vi "VisualizeStatus.vi"() -> ()   [LabVIEW 2017, in "Visualization.lvlib" / "VisualizeStatus.lvclass"]
uses:
  VisualizeStatus.lvclass
  Framework/Bus_class/Bus.lvclass
  VisializeBase_class/Typedefs/VisualizeData.ctl
  VisializeBase_class/Typedefs/clVisualizeData.ctl
  Modules/EventPlugins/EventPluginBaseClass/TypeDefs/clEvtReportArray.ctl
  Modules/EventPlugins/EventPluginBaseClass/TypeDefs/clEvtReport.ctl
  Modules/EventPlugins/EventPluginBaseClass/TypeDefs/dblEvtSignalArray.ctl
  Modules/NetworkImpairmentModule/PublicAPI/Arguments/Broadcasts/dblNetworkTime.ctl
  Modules/NetworkImpairmentModule/PublicAPI/Arguments/Broadcasts/dblPktLoss.ctl
  Modules/FlagImpairModule/PublicAPI/Arguments/Broadcasts/ui32FlagImpairmentArray.ctl
  Framework/Bus_class/Broadcast/Typedefs/clDidInit.ctl
  Modules/EventModule/PublicAPI/Arguments/Broadcasts/clStatUpdate.ctl
  VisializeBase_class/Requests/clUserEventType.ctl
  <vilib>/event_ctls.llb/usereventprio.ctl
  <vilib>/Utility/miscctls.llb/LVStringsAndValuesArrayTypeDef_U8.ctl
  QMH/Typedefs/clEvtRptArray.ctl
  QMH/Typedefs/clPmuImpairRptArray.ctl
  QMH/Typedefs/clNetImpairmentTime.ctl
  QMH/Typedefs/clNetIPktLoss.ctl
  QMH/Typedefs/clFlagImpairArray.ctl
  QMH/Typedefs/clEvtRptSignal.ctl
  <vilib>/Utility/error.llb/Error Cluster From Error Code.vi
  <vilib>/ErrorRing/Error Ring.xnode
  VisializeBase_class/VisualizeBase_class.lvclass
  <userlib>/NIST/NISTErrorLib/NISTErrorLib.lvlib
  Framework/Bus_class/Bus_class.lvlib
  Modules/EventModule/EventModule.lvlib
  Modules/PmuImpairModule/PmuImpairModule.lvlib
  Modules/NetworkImpairmentModule/NetworkImpairmentModule.lvlib
  Modules/FlagImpairModule/FlagImpairModule.lvlib
  Modules/EventPlugins/EventPluginBaseClass/EventPluginBaseClass.lvclass
  VisualizeApp_class/VisualizeAppBase_class.lvclass
panel:
  in  "btnClear":bool
  out "Status Log":string
  in  "QueName":string="BaseVisQue"
  in  "Bus Number":u8(ring)
  out "ErrorArray":errorcluster[](array[cluster])
  in  "btnStop":bool
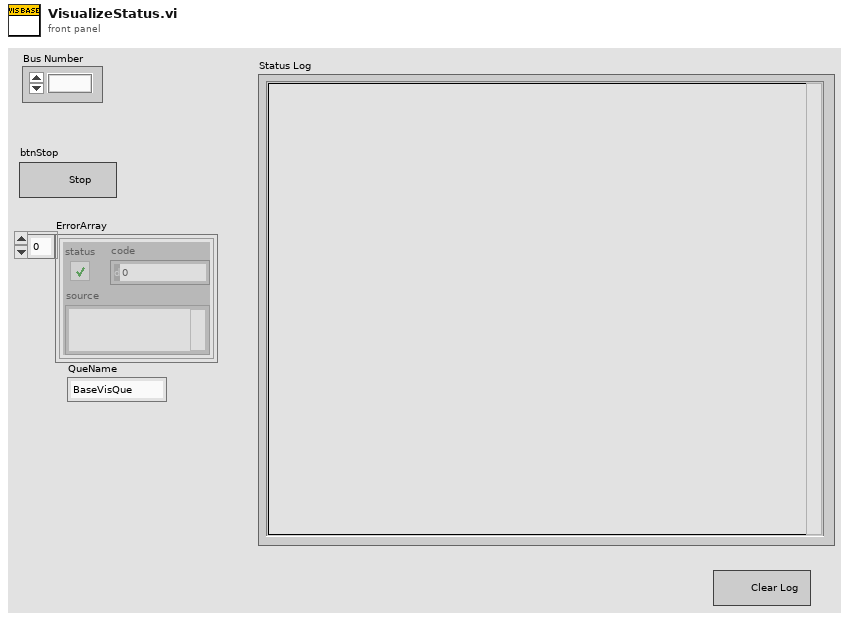
[diagram p1: front panel]
types:
  T1 = typedef "Visualization.lvlib/VisualizeBase_class.lvclass/VisualizeData.ctl" = T2[]
  T2 = typedef "Visualization.lvlib/VisualizeAppBase_class.lvclass/clVisualizeData.ctl" = cluster{"clEvtReportArray":T3, "dblEventSignalArray":T5, "clPmuImpairRptArray":T3, "dblNetworkTime":T6, "dblPktLoss":T7, "FlagImpairArray":T8, "TimeArray":dbl[]}
  T3 = typedef "EventPlugins.lvlib/EventPluginBaseClass.lvclass/clEvtReportArray.ctl" = T4[]
  T4 = typedef "EventPlugins.lvlib/EventPluginBaseClass.lvclass/clEvtReport.ctl" = cluster{"Timestamp":dbl, "Synx":cdb[], "Freq":dbl, "ROCOF":dbl, "ID":i16}
  T5 = typedef "EventPlugins.lvlib/EventPluginBaseClass.lvclass/dblEvtSignalArray.ctl" = dbl[][]
  T6 = typedef "NetworkImpairmentModule.lvlib/dblNetworkTime.ctl" = dbl[]
  T7 = typedef "NetworkImpairmentModule.lvlib/dblPktLoss.ctl" = dbl[]
  T8 = typedef "FlagImpairModule.lvlib/ui32FlagImpairmentArray.ctl" = u32[]
  T9 = typedef "Visualization.lvlib/VisualizeBase_class.lvclass/clRequestEvents.ctl" = cluster{"StopRequest":refnum<user-event>}
  T10 = typedef "Bus_class.lvlib/clBroadcastEvents.ctl" = cluster{"DidInit":refnum<user-event>, "DidStop":refnum<user-event>}
  T11 = typedef "EventModule.lvlib/clBroadcastEvents.ctl" = cluster{"DidInit":refnum<user-event>, "StatusUpdate":refnum<user-event>, "ErrorReport":refnum<user-event>, "DidStop":refnum<user-event>, "ReadEvtConfig":refnum<user-event>, "ReadTimeArray":refnum<user-event>, "ReadEvtParams":refnum<user-event>, "GetEvtReportArray":refnum<user-event>, "ReadPathToPlugin":refnum<user-event>, "GetEvtSignal":refnum<user-event>, "ReadBusNumber":refnum<user-event>}
  T12 = typedef "PmuImpairModule.lvlib/clBroadcastEvents.ctl" = cluster{"DidInit":refnum<user-event>, "StatusUpdate":refnum<user-event>, "ErrorReport":refnum<user-event>, "DidStop":refnum<user-event>, "ImpairConfig":refnum<user-event>, "ImpairParams":refnum<user-event>, "ImpairReports":refnum<user-event>, "PathToPlugin":refnum<user-event>, "BusNumber":refnum<user-event>}
  T13 = typedef "NetworkImpairmentModule.lvlib/clBroadcastEvents.ctl" = cluster{"DidInit":refnum<user-event>, "StatusUpdate":refnum<user-event>, "ErrorReport":refnum<user-event>, "DidStop":refnum<user-event>, "ReadNetImpParams":refnum<user-event>, "ReadLossThreshold":refnum<user-event>, "GetNetworkTime":refnum<user-event>, "GetPktLoss":refnum<user-event>, "ReadPathToPlugin":refnum<user-event>}
  T14 = typedef "FlagImpairModule.lvlib/clBroadcastEvents.ctl" = cluster{"DidInit":refnum<user-event>, "StatusUpdate":refnum<user-event>, "ErrorReport":refnum<user-event>, "DidStop":refnum<user-event>, "ReadFlagImpairConfig":refnum<user-event>, "ReadPluginINIFilePath":refnum<user-event>, "ReadFlagImpairParams":refnum<user-event>, "ReadTimeArray":refnum<user-event>, "GetFlagImpairment":refnum<user-event>}
  T15 = typedef "LVStringsAndValuesArrayTypeDef_U8.ctl" = cluster{"String":string, "Value":u8}[]
  T16 = typedef "Visualization.lvlib/VisualizeBase_class.lvclass/clEvtRptArray.ctl" = cluster{"BusIndex":i32, "clImpairReportArray":T3}
  T17 = typedef "EventModule.lvlib/clStatUpdate.ctl" = cluster{"Status":string}
  T18 = typedef "Visualization.lvlib/VisualizeBase_class.lvclass/clPmuImpairRptArray.ctl" = cluster{"BusIndex":i32, "clImpairReportArray":T3}
  T19 = typedef "Visualization.lvlib/VisualizeBase_class.lvclass/clNetImpairmentTime.ctl" = cluster{"BusIndex":i32, "clNetImpairTimeArray":T6}
  T20 = typedef "Visualization.lvlib/VisualizeBase_class.lvclass/clNetIPktLoss.ctl" = cluster{"BusIndex":i32, "clNetPktLoss":T7}
  T21 = typedef "Visualization.lvlib/VisualizeBase_class.lvclass/clFlagImpairArray.ctl" = cluster{"BusIndex":i32, "FlagImpairArray":T8}
  T22 = typedef "Visualization.lvlib/VisualizeBase_class.lvclass/clEvtRptSignal.ctl" = cluster{"BusIndex":i32, "dblEventSignalArray":T5}
  T23 = typedef "Visualization.lvlib/VisualizeBase_class.lvclass/clUserEventType.ctl" = cluster{"BusIndex":i8, "Data":variant}
  T24 = typedef "usereventprio.ctl" = enum32{"high priority", "normal priority"}
  T25 = typedef "Bus_class.lvlib/clDidInit.ctl" = cluster{"Bus":refnum<vi>, "Init?":bool}
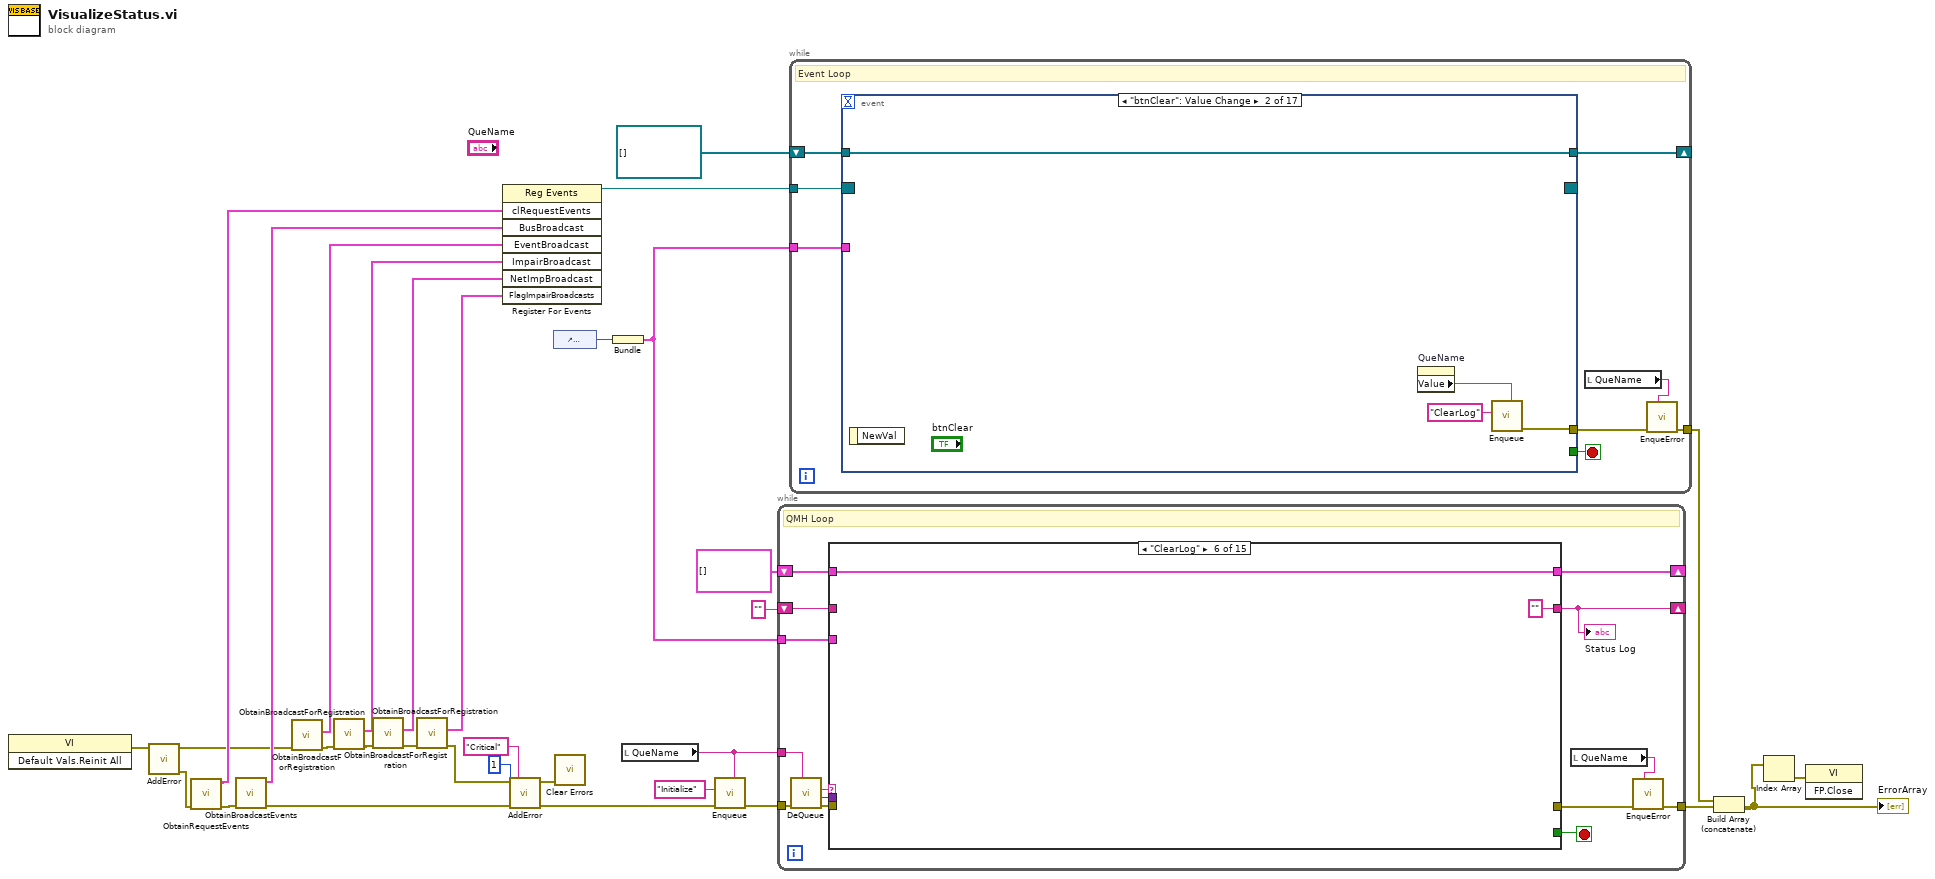
[diagram p0: block diagram]
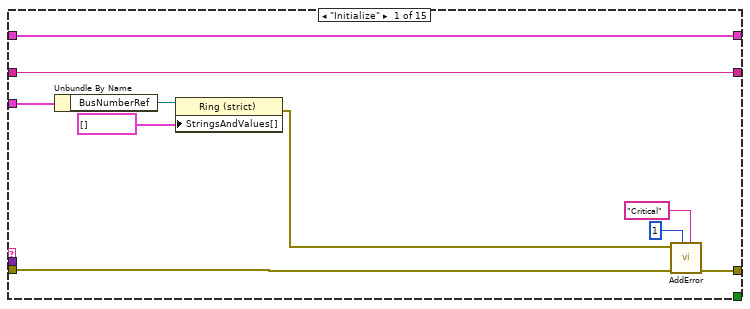
[diagram p2: hidden frame]
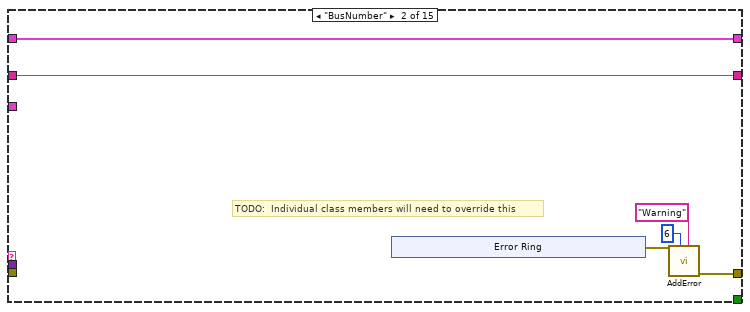
[diagram p3: hidden frame]
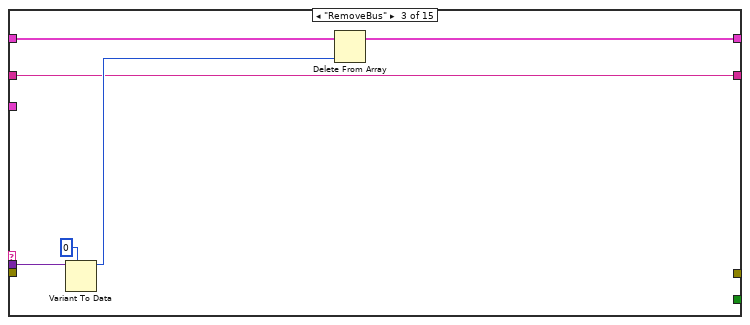
[diagram p4: hidden frame]
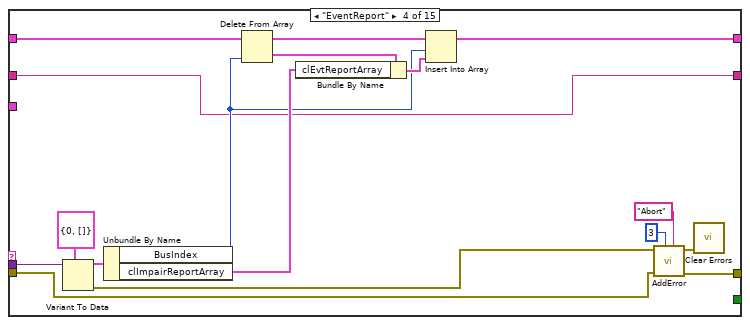
[diagram p5: hidden frame]
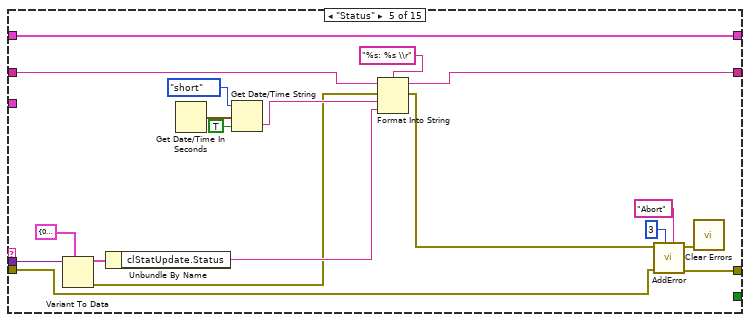
[diagram p6: hidden frame]
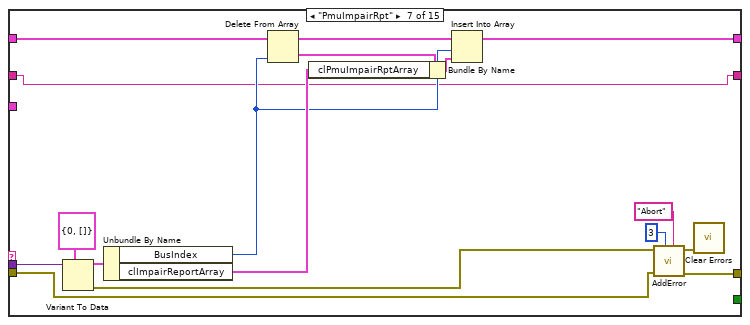
[diagram p7: hidden frame]
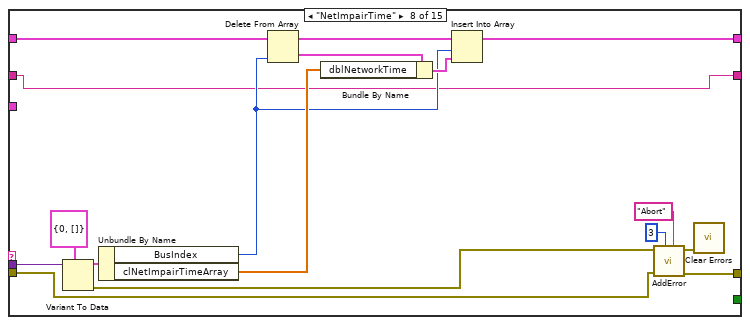
[diagram p8: hidden frame]
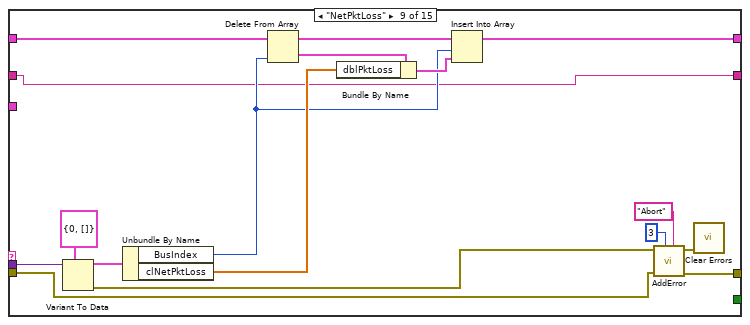
[diagram p9: hidden frame]
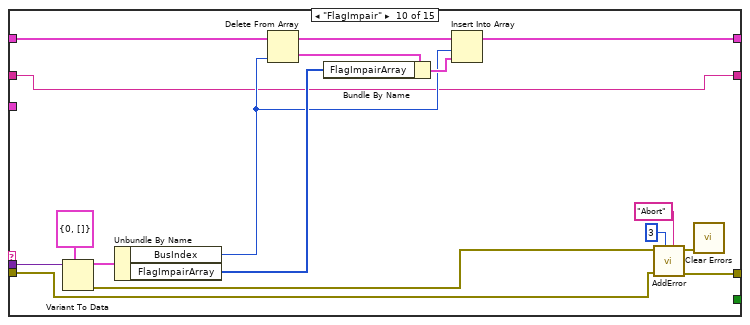
[diagram p10: hidden frame]
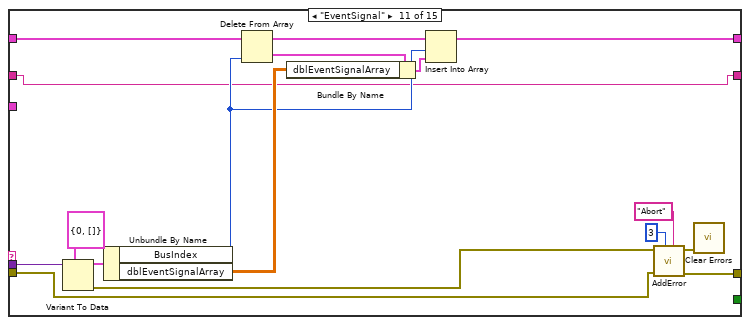
[diagram p11: hidden frame]
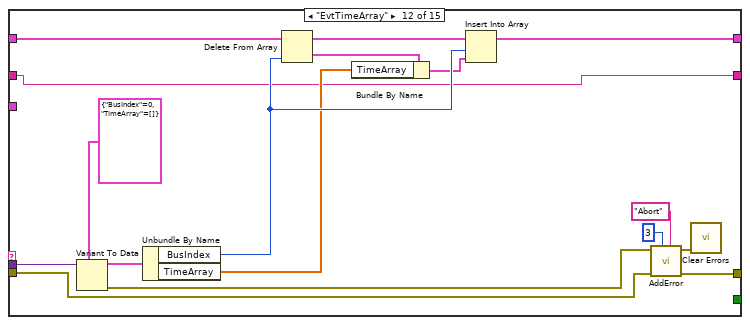
[diagram p12: hidden frame]
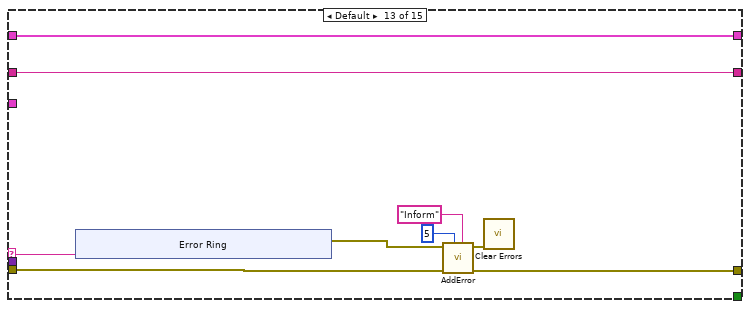
[diagram p13: hidden frame]
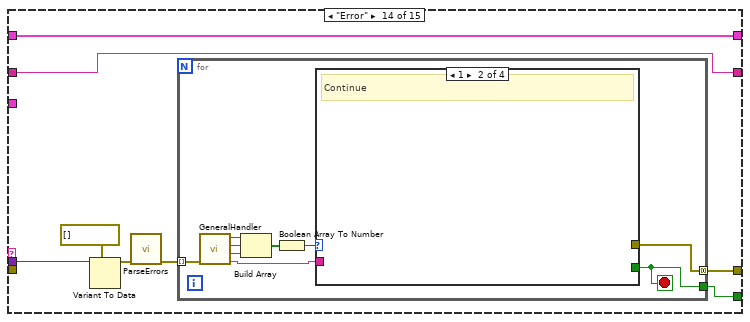
[diagram p14: hidden frame]
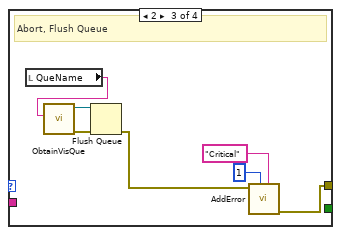
[diagram p16: hidden frame]
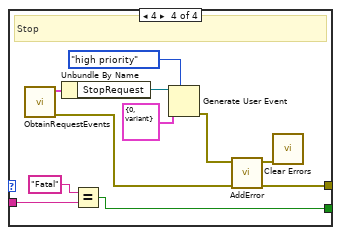
[diagram p17: hidden frame]
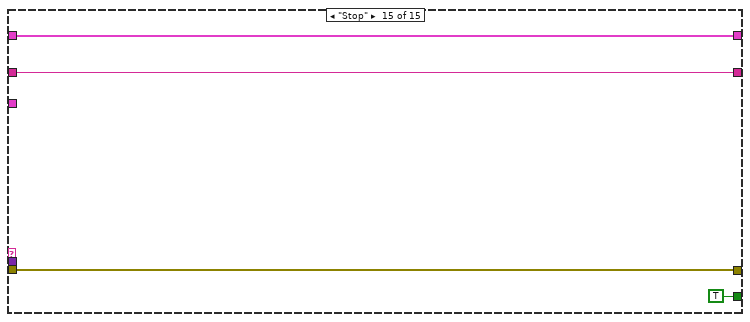
[diagram p18: hidden frame]
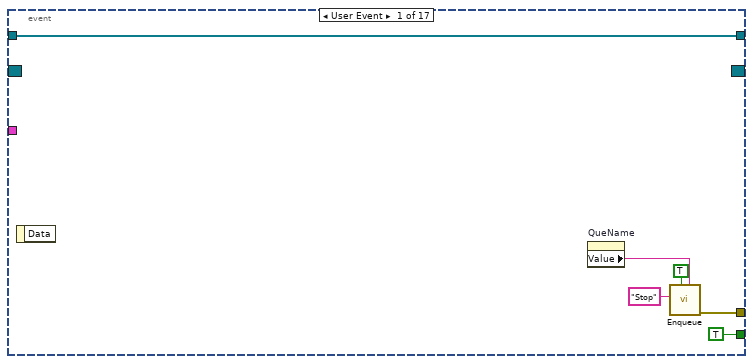
[diagram p19: hidden frame]
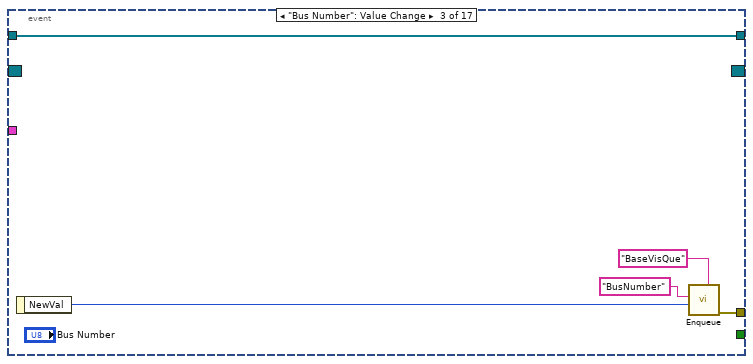
[diagram p20: hidden frame]
diagram:
  n1 = invoke class="VI" method="Default Vals.Reinit All"() -> (error out=w22:errorcluster)  [unwired: 3 in, 2 out]
  n2 = call <userlib>:"AddError.vi"("error in (no error)"=w22) -> ("ErrorArray"=w21:errorcluster[], "error out"=w13:errorcluster)  [unwired: 9 in]
  n3 = call "ObtainRequestEvents.vi"("Error"=w21) -> ("Error"=w26:errorcluster[], "clRequestEvents"=w30:T9)  [unwired: 9 in]
  n4 = call "ObtainBroadcastEvents.vi"("ErrorArray"=w26) -> ("ErrorArray"=w12:errorcluster[], "BusBroadcast"=w25:T10)  [unwired: 9 in]
  n5 = call "ObtainBroadcastForRegistration.vi"("error in (no error)"=w13) -> ("error out"=w16:errorcluster, "EventBroadcast"=w20:T11)  [unwired: 9 in]
  n6 = call "ObtainBroadcastForRegistration.vi"("error in (no error)"=w16) -> ("error out"=w15:errorcluster, "ImpairBroadcast"=w19:T12)  [unwired: 9 in]
  n7 = call "ObtainBroadcastForRegistration.vi"("error in (no error)"=w15) -> ("error out"=w14:errorcluster, "NetImpBroadcast"=w18:T13)  [unwired: 9 in]
  n8 = call "ObtainBroadcastForRegistration.vi"("error in (no error)"=w14) -> ("error out"=w11:errorcluster, "FlagImpairBroadcasts"=w17:T14)  [unwired: 9 in]
  n9 = register-events(w30, w25, w20, w19, w18, w17) -> (reference out=w29:refnum<event-registration>)  [unwired: 2 in, 1 out]
  n10 = call <userlib>:"AddError.vi"("Severity"="Critical" ("String"), "Priority"=u8 1, "ErrorArray"=w12, "error in (no error)"=w11) -> ("ErrorArray"=w8:errorcluster[], "error out"=w5:errorcluster)  [unwired: 6 in]
  n11 = control-ref of="BusNumberRef"() -> (w24:refnum<vi>)
  n12 = call <vilib>:"Clear Errors.vi"("error in (no error)"=w5) -> ()  [unwired: 5 in, 2 out]
  n13 = Bundle("BusNumberRef"=w24) -> (w6:cluster{"BusNumberRef":refnum<vi>})  [unwired: 1 in]
  n14 = local read "QueName"() -> (w4:string)
  n15 = call "Enqueue.vi"("QueName"=w4, "Error"=w8, "Message"="Initialize") -> ("Error"=w31:errorcluster[])  [unwired: 8 in]
  n16 = while {
    tunnel: w31 -> [w46]
    tunnel: [w40] -> w28
    tunnel: w6 -> [w39]
    shift-right: [w37] -> _
    shift-left: T1 [] ("VisualizeData") -> [w38]
    tunnel: w4 -> [w35]
    shift-right: [w33] -> _
    shift-left: "" -> [w34]
    stop <- w41 stop-if-true
    # "QMH Loop"
    n17 = call "DeQueue.vi"("QueName"=w35, "Error"=w46) -> ("Error"=w43:errorcluster[], "Data"=w44:variant, "Message"=w45:string)  [unwired: 7 in]
    n18 = case shown="\"ClearLog\"" w45 {
      selector: w45 -> [_ _ _ _ _ _ _ _ _ _ _ _ w222 _ _]
      tunnel: w44 -> [_ _ w73 w90 w109 _ w128 w145 w162 w179 w196 w204 _ w237 _]
      tunnel: w43 -> [w53 _ _ w75 w103 _ w113 w130 w147 w164 w181 w198 w220 _ w267]
      tunnel: [w52 w62 _ w80 w107 _ w118 w135 w152 w169 w186 w200 w219 w233 w267] -> w42
      tunnel: [_ _ _ _ _ _ _ _ _ _ _ _ _ w232 TRUE] -> w41
      tunnel: w39 -> [w56 _ _ _ _ _ _ _ _ _ _ _ _ _ _]
      tunnel: w38 -> [w48 w58 w71 w86 w102 w110 w124 w141 w158 w175 w192 w206 w215 w231 w266]
      tunnel: [w48 w58 w70 w87 w102 w110 w125 w142 w159 w176 w193 w205 w215 w231 w266] -> w37
      tunnel: w34 -> [w47 w57 w68 w74 w96 _ w112 w129 w146 w163 w180 w197 w214 w230 w265]
      tunnel: [w47 w57 w68 w74 w95 "" w112 w129 w146 w163 w180 w197 w214 w230 w265] -> w33
      frame "Initialize" {
        n19 = Unbundle By Name(w56) -> ("BusNumberRef"=w55:refnum<vi>)
        n20 = property class="Ring (strict)"(reference=w55, "StringsAndValues[]"=T15 [] ("Strings And Values []")) -> (error out=w51:errorcluster)  [unwired: 1 in, 1 out]
        n21 = call <userlib>:"AddError.vi"("Severity"="Critical" ("String"), "Priority"=u8 1, "ErrorArray"=w53, "error in (no error)"=w51) -> ("ErrorArray"=w52:errorcluster[])  [unwired: 6 in, 1 out]
      }
      frame "BusNumber" {
        # "TODO:  Individual class members will need to override this"
        n22 = xnode "Error Ring"() -> ("error out"=w61:errorcluster)
        n23 = call <userlib>:"AddError.vi"("Severity"="Warning" ("String"), "Priority"=u8 6, "error in (no error)"=w61) -> ("ErrorArray"=w62:errorcluster[])  [unwired: 7 in, 1 out]
      }
      frame "RemoveBus" {
        n24 = Variant To Data(type=0, Variant=w73) -> (data=w69:i32)  [unwired: 1 in, 1 out]
        n25 = Delete From Array(array=w71, index=w69) -> (array with subset deleted=w70:T1)  [unwired: 1 in, 1 out]
      }
      frame "EventReport" {
        n26 = Variant To Data(type=T16 {"BusIndex"=0, "clImpairReportArray"=[]} ("clEvtReportArray"), Variant=w90) -> (data=w88:T16, error out=w79:errorcluster)  [unwired: 1 in]
        n27 = Unbundle By Name(w88) -> ("BusIndex"=w81:i32, "clImpairReportArray"=w83:T3)
        n28 = Delete From Array(array=w86, index=w81) -> (deleted portion=w84:T2, array with subset deleted=w85:T1)  [unwired: 1 in]
        n29 = Bundle By Name(cluster=w84, "clEvtReportArray"=w83) -> (w82:T2)
        n30 = Insert Into Array(array=w85, index=w81, new element=w82) -> (w87:T1)
        n31 = call <userlib>:"AddError.vi"("Severity"="Abort" ("String"), "Priority"=u8 3, "ErrorArray"=w75, "error in (no error)"=w79) -> ("ErrorArray"=w80:errorcluster[], "error out"=w78:errorcluster)  [unwired: 6 in]
        n32 = call <vilib>:"Clear Errors.vi"("error in (no error)"=w78) -> ()  [unwired: 5 in, 2 out]
      }
      frame "Status" {
        n33 = Variant To Data(type=cluster{i32, "clStatUpdate":T17} {0, "clStatUpdate"={"Status"=""}} ("output cluster"), Variant=w109) -> (data=w108:cluster{i32, "clStatUpdate":T17}, error out=w93:errorcluster)  [unwired: 1 in]
        n34 = Unbundle By Name(w108) -> ("clStatUpdate.Status"=w94:string)
        n35 = Get Date/Time In Seconds() -> (seconds since 1Jan1904=w98:timestamp)
        n36 = Get Date/Time String(date format (0)=enum16{"short", "long", "abbreviated"}."short", seconds (now)=w98, want seconds? (F)=TRUE) -> (time string=w101:string)  [unwired: 1 out]
        n37 = Format Into String(format string="%s: %s \\r", initial string=w96, error in=w93, w101, w94) -> (resulting string=w95:string, error out=w92:errorcluster)
        n38 = call <userlib>:"AddError.vi"("Severity"="Abort" ("String"), "Priority"=u8 3, "ErrorArray"=w103, "error in (no error)"=w92) -> ("ErrorArray"=w107:errorcluster[], "error out"=w106:errorcluster)  [unwired: 6 in]
        n39 = call <vilib>:"Clear Errors.vi"("error in (no error)"=w106) -> ()  [unwired: 5 in, 2 out]
      }
      frame "ClearLog" {
      }
      frame "PmuImpairRpt" {
        n40 = Variant To Data(type=T18 {"BusIndex"=0, "clImpairReportArray"=[]} ("clImpairReportArray"), Variant=w128) -> (data=w126:T18, error out=w117:errorcluster)  [unwired: 1 in]
        n41 = Unbundle By Name(w126) -> ("BusIndex"=w119:i32, "clImpairReportArray"=w121:T3)
        n42 = Delete From Array(array=w124, index=w119) -> (deleted portion=w122:T2, array with subset deleted=w123:T1)  [unwired: 1 in]
        n43 = Bundle By Name(cluster=w122, "clPmuImpairRptArray"=w121) -> (w120:T2)
        n44 = Insert Into Array(array=w123, index=w119, new element=w120) -> (w125:T1)
        n45 = call <userlib>:"AddError.vi"("Severity"="Abort" ("String"), "Priority"=u8 3, "ErrorArray"=w113, "error in (no error)"=w117) -> ("ErrorArray"=w118:errorcluster[], "error out"=w116:errorcluster)  [unwired: 6 in]
        n46 = call <vilib>:"Clear Errors.vi"("error in (no error)"=w116) -> ()  [unwired: 5 in, 2 out]
      }
      frame "NetImpairTime" {
        n47 = Variant To Data(type=T19 {"BusIndex"=0, "clNetImpairTimeArray"=[]} ("clImpairReportArray"), Variant=w145) -> (data=w143:T19, error out=w134:errorcluster)  [unwired: 1 in]
        n48 = Unbundle By Name(w143) -> ("BusIndex"=w136:i32, "clNetImpairTimeArray"=w138:T6)
        n49 = Delete From Array(array=w141, index=w136) -> (deleted portion=w139:T2, array with subset deleted=w140:T1)  [unwired: 1 in]
        n50 = Bundle By Name(cluster=w139, "dblNetworkTime"=w138) -> (w137:T2)
        n51 = Insert Into Array(array=w140, index=w136, new element=w137) -> (w142:T1)
        n52 = call <userlib>:"AddError.vi"("Severity"="Abort" ("String"), "Priority"=u8 3, "ErrorArray"=w130, "error in (no error)"=w134) -> ("ErrorArray"=w135:errorcluster[], "error out"=w133:errorcluster)  [unwired: 6 in]
        n53 = call <vilib>:"Clear Errors.vi"("error in (no error)"=w133) -> ()  [unwired: 5 in, 2 out]
      }
      frame "NetPktLoss" {
        n54 = Variant To Data(type=T20 {"BusIndex"=0, "clNetPktLoss"=[]} ("clNetPktLoss"), Variant=w162) -> (data=w160:T20, error out=w151:errorcluster)  [unwired: 1 in]
        n55 = Unbundle By Name(w160) -> ("BusIndex"=w153:i32, "clNetPktLoss"=w155:T7)
        n56 = Delete From Array(array=w158, index=w153) -> (deleted portion=w156:T2, array with subset deleted=w157:T1)  [unwired: 1 in]
        n57 = Bundle By Name(cluster=w156, "dblPktLoss"=w155) -> (w154:T2)
        n58 = Insert Into Array(array=w157, index=w153, new element=w154) -> (w159:T1)
        n59 = call <userlib>:"AddError.vi"("Severity"="Abort" ("String"), "Priority"=u8 3, "ErrorArray"=w147, "error in (no error)"=w151) -> ("ErrorArray"=w152:errorcluster[], "error out"=w150:errorcluster)  [unwired: 6 in]
        n60 = call <vilib>:"Clear Errors.vi"("error in (no error)"=w150) -> ()  [unwired: 5 in, 2 out]
      }
      frame "FlagImpair" {
        n61 = Variant To Data(type=T21 {"BusIndex"=0, "FlagImpairArray"=[]} ("clFlagImpairArray"), Variant=w179) -> (data=w177:T21, error out=w168:errorcluster)  [unwired: 1 in]
        n62 = Unbundle By Name(w177) -> ("BusIndex"=w170:i32, "FlagImpairArray"=w172:T8)
        n63 = Delete From Array(array=w175, index=w170) -> (deleted portion=w173:T2, array with subset deleted=w174:T1)  [unwired: 1 in]
        n64 = Bundle By Name(cluster=w173, "FlagImpairArray"=w172) -> (w171:T2)
        n65 = Insert Into Array(array=w174, index=w170, new element=w171) -> (w176:T1)
        n66 = call <userlib>:"AddError.vi"("Severity"="Abort" ("String"), "Priority"=u8 3, "ErrorArray"=w164, "error in (no error)"=w168) -> ("ErrorArray"=w169:errorcluster[], "error out"=w167:errorcluster)  [unwired: 6 in]
        n67 = call <vilib>:"Clear Errors.vi"("error in (no error)"=w167) -> ()  [unwired: 5 in, 2 out]
      }
      frame "EventSignal" {
        n68 = Variant To Data(type=T22 {"BusIndex"=0, "dblEventSignalArray"=[]} ("clEvtReportArray"), Variant=w196) -> (data=w194:T22, error out=w185:errorcluster)  [unwired: 1 in]
        n69 = Unbundle By Name(w194) -> ("BusIndex"=w187:i32, "dblEventSignalArray"=w189:T5)
        n70 = Delete From Array(array=w192, index=w187) -> (deleted portion=w190:T2, array with subset deleted=w191:T1)  [unwired: 1 in]
        n71 = Bundle By Name(cluster=w190, "dblEventSignalArray"=w189) -> (w188:T2)
        n72 = Insert Into Array(array=w191, index=w187, new element=w188) -> (w193:T1)
        n73 = call <userlib>:"AddError.vi"("Severity"="Abort" ("String"), "Priority"=u8 3, "ErrorArray"=w181, "error in (no error)"=w185) -> ("ErrorArray"=w186:errorcluster[], "error out"=w184:errorcluster)  [unwired: 6 in]
        n74 = call <vilib>:"Clear Errors.vi"("error in (no error)"=w184) -> ()  [unwired: 5 in, 2 out]
      }
      frame "EvtTimeArray" {
        n75 = Variant To Data(type=cluster{"BusIndex":i32, "TimeArray":dbl[]} {"BusIndex"=0, "TimeArray"=[]} ("cluster"), Variant=w204) -> (data=w207:cluster{"BusIndex":i32, "TimeArray":dbl[]}, error out=w199:errorcluster)  [unwired: 1 in]
        n76 = Unbundle By Name(w207) -> ("BusIndex"=w212:i32, "TimeArray"=w210:dbl[])
        n77 = Delete From Array(array=w206, index=w212) -> (deleted portion=w209:T2, array with subset deleted=w208:T1)  [unwired: 1 in]
        n78 = Bundle By Name(cluster=w209, "TimeArray"=w210) -> (w211:T2)
        n79 = Insert Into Array(array=w208, index=w212, new element=w211) -> (w205:T1)
        n80 = call <userlib>:"AddError.vi"("Severity"="Abort" ("String"), "Priority"=u8 3, "ErrorArray"=w198, "error in (no error)"=w199) -> ("ErrorArray"=w200:errorcluster[], "error out"=w201:errorcluster)  [unwired: 6 in]
        n81 = call <vilib>:"Clear Errors.vi"("error in (no error)"=w201) -> ()  [unwired: 5 in, 2 out]
      }
      frame Default {
        n82 = xnode "Error Ring"("parameter 0"=w222) -> ("error out"=w221:errorcluster)
        n83 = call <userlib>:"AddError.vi"("Severity"="Inform" ("String"), "Priority"=u8 5, "ErrorArray"=w220, "error in (no error)"=w221) -> ("ErrorArray"=w219:errorcluster[], "error out"=w218:errorcluster)  [unwired: 6 in]
        n84 = call <vilib>:"Clear Errors.vi"("error in (no error)"=w218) -> ()  [unwired: 5 in, 2 out]
      }
      frame "Error" {
        n85 = Variant To Data(type=errorcluster[] [], Variant=w237) -> (data=w235:errorcluster[])  [unwired: 1 in, 1 out]
        n86 = call <userlib>:"ParseErrors.vi"("ErrorArray"=w235) -> ("ErrorArray"=w234:errorcluster[])  [unwired: 8 in, 2 out]
        n87 = for {
          tunnel: w234 -> [w246] mode=indexing
          tunnel: [w240] -> w233 mode=concatenating
          tunnel: [w238] -> w232
          stop <- w238 stop-if-true
          n88 = call <userlib>:"GeneralHandler.vi"("error in (no error)"=w246) -> ("Severity"=w239:string, "Stop"=w243:bool, "Abort"=w244:bool, "Continue"=w245:bool)  [unwired: 7 in]
          n89 = Build Array(w245, w244, w243) -> (w242:bool[])
          n90 = Boolean Array To Number(Boolean array=w242) -> (number=w241:u32)
          n91 = case shown="1" w241 {
            tunnel: [_ _ w251 w262] -> w240
            tunnel: w239 -> [_ _ _ w256]
            tunnel: [_ _ _ w254] -> w238
            frame 0, Default {
              # "No Dialog"
            }
            frame 1 {
              # "Continue"
            }
            frame 2 {
              # "Abort, Flush Queue"
              n92 = local read "QueName"() -> (w247:string)
              n93 = call "ObtainVisQue.vi"("QueName"=w247) -> ("error out"=w253:errorcluster, "queue out"=w252:refnum<queue>)  [unwired: 9 in]
              n94 = Flush Queue(queue=w252, error in (no error)=w253) -> (error out=w250:errorcluster)  [unwired: 2 out]
              n95 = call <userlib>:"AddError.vi"("Severity"="Critical" ("String"), "Priority"=u8 1, "error in (no error)"=w250) -> ("ErrorArray"=w251:errorcluster[])  [unwired: 7 in, 1 out]
            }
            frame 4 {
              # "Stop"
              n96 = call "ObtainRequestEvents.vi"() -> ("Error"=w260:errorcluster[], "clRequestEvents"=w264:T9)  [unwired: 10 in]
              n97 = Unbundle By Name(w264) -> ("StopRequest"=w263:refnum<user-event>)
              n98 = Equal?(x="Fatal", y=w256) -> (x = y?=w254:bool)
              n99 = Generate User Event(priority (normal)=usereventprio."high priority", user event=w263, event data cluster=T23 {"BusIndex"=0, "Data"=variant} ("event data")) -> (error out=w261:errorcluster)  [unwired: 1 in, 1 out]
              n100 = call <userlib>:"AddError.vi"("ErrorArray"=w260, "error in (no error)"=w261) -> ("ErrorArray"=w262:errorcluster[], "error out"=w257:errorcluster)  [unwired: 8 in]
              n101 = call <vilib>:"Clear Errors.vi"("error in (no error)"=w257) -> ()  [unwired: 5 in, 2 out]
            }
          }
        }
      }
      frame "Stop" {
      }
    }
    "Status Log" <- w33
    n102 = local read "QueName"() -> (w36:string)
    n103 = call "EnqueError.vi"("QueName"=w36, "Error"=w42) -> ("Error"=w40:errorcluster[])  [unwired: 9 in]
  }
  n104 = while {
    tunnel: w29 -> [w276]
    tunnel: [w273] -> w27
    tunnel: w6 -> [w272]
    shift-right: [w270] -> _
    shift-left: refnum<class "Bus.lvclass">[] [] -> [w271]
    stop <- w275 stop-if-true
    # "Event Loop"
    n105 = event shown="[1] \"btnClear\": Value Change" {
      selector: w276 -> [_ _ _ _ _ _ _ _ _ _ _ _ _ _ _ _ _]
      dyn-events: [_ _ _ w300 _ _ _ _ _ _ _ _ _ _ _ _ _] -> _
      timeout: _ -> [_ _ _ _ _ _ _ _ _ _ _ _ _ _ _ _ _]
      tunnel: [TRUE _ _ _ _ _ _ _ _ _ _ _ _ _ _ _ _] -> w275
      tunnel: [w281 w285 w291 w303 w321 w327 w355 w383 w411 w439 w468 w491 w514 w537 w560 w583 w610] -> w274
      tunnel: w272 -> [_ _ _ w313 w325 _ _ _ _ _ _ _ _ _ _ _ _]
      tunnel: w271 -> [w278 w286 w288 w312 w324 w328 w356 w384 w412 w440 w471 w494 w517 w540 w563 w586 w604]
      tunnel: [w278 w286 w288 w309 w323 w326 w354 w382 w410 w438 w466 w489 w512 w535 w558 w581 w604] -> w270
      event User Event {
        n106 = event-data() -> ()  [unwired: 1 in, 1 out]
        n107 = property on="QueName" class="Str"() -> ("Value"=w277:string)  [unwired: 2 in, 2 out]
        n108 = call "Enqueue.vi"("QueName"=w277, "Priority? (F)"=TRUE, "Message"="Stop") -> ("Error"=w281:errorcluster[])  [unwired: 8 in]
      }
      event "btnClear": Value Change {
        n109 = event-data() -> ()  [unwired: 1 in, 1 out]
        n110 = property on="QueName" class="Str"() -> ("Value"=w284:string)  [unwired: 2 in, 2 out]
        n111 = call "Enqueue.vi"("QueName"=w284, "Message"="ClearLog") -> ("Error"=w285:errorcluster[])  [unwired: 9 in]
      }
      event "Bus Number": Value Change {
        n112 = event-data() -> ("NewVal"=w290:u8)  [unwired: 1 in]
        n113 = call "Enqueue.vi"("QueName"="BaseVisQue", "Data"=w290, "Message"="BusNumber") -> ("Error"=w291:errorcluster[])  [unwired: 8 in]
      }
      event User Event {
        n114 = event-data() -> ("Data"=w316:variant)  [unwired: 1 in]
        n115 = Unbundle By Name(w313) -> ("BusNumberRef"=w311:refnum<vi>)
        n116 = Variant To Data(type=T25 {"Bus"=refnum, "Init?"=FALSE} ("clBusDidInit"), Variant=w316) -> (data=w314:T25)  [unwired: 1 in, 1 out]
        n117 = Unbundle By Name(w314) -> ("Bus"=w310:refnum<vi>)
        n118 = call "AddBus.vi"("BusRef"=w310, "BusNumberRef"=w311, "BusArray"=w312) -> ("BusArray"=w309:refnum<class "Bus.lvclass">[])  [unwired: 8 in]
        n119 = call "ObtainRequestEvents.vi"() -> ("Error"=w295:errorcluster[], "clRequestEvents"=w293:T9)  [unwired: 10 in]
        n120 = call "ObtainBroadcastEvents.vi"("ErrorArray"=w295) -> ("ErrorArray"=w294:errorcluster[], "BusBroadcast"=w292:T10)  [unwired: 9 in]
        n121 = call "ObtainBroadcastForRegistration.vi"() -> ("error out"=w308:errorcluster, "EventBroadcast"=w299:T11)  [unwired: 10 in]
        n122 = call "ObtainBroadcastForRegistration.vi"("error in (no error)"=w308) -> ("error out"=w307:errorcluster, "ImpairBroadcast"=w298:T12)  [unwired: 9 in]
        n123 = call "ObtainBroadcastForRegistration.vi"("error in (no error)"=w307) -> ("error out"=w306:errorcluster, "NetImpBroadcast"=w297:T13)  [unwired: 9 in]
        n124 = call "ObtainBroadcastForRegistration.vi"("error in (no error)"=w306) -> ("error out"=w301:errorcluster, "FlagImpairBroadcasts"=w296:T14)  [unwired: 9 in]
        n125 = register-events(w293, w292, w299, w298, w297, w296) -> (reference out=w300:refnum<event-registration>)  [unwired: 2 in, 1 out]
        n126 = call <userlib>:"AddError.vi"("Severity"="Critical" ("String"), "Priority"=u8 1, "ErrorArray"=w294, "error in (no error)"=w301) -> ("ErrorArray"=w303:errorcluster[], "error out"=w302:errorcluster)  [unwired: 6 in]
        n127 = call <vilib>:"Clear Errors.vi"("error in (no error)"=w302) -> ()  [unwired: 5 in, 2 out]
      }
      event User Event {
        n128 = event-data() -> ("BusNumber"=w318:i8)  [unwired: 1 in]
        n129 = Unbundle By Name(w325) -> ("BusNumberRef"=w322:refnum<vi>)
        n130 = call "RemoveBus.vi"("BusArray"=w324, "BusNumberRef"=w322, "BusNumber"=w318) -> ("BusArray"=w323:refnum<class "Bus.lvclass">[], "BusIndex"=w320:i32)  [unwired: 6 in]
        n131 = call "Enqueue.vi"("QueName"="BaseVisQue", "Data"=w320, "Message"="RemoveBus") -> ("Error"=w321:errorcluster[])  [unwired: 8 in]
      }
      event User Event {
        w329 = FALSE  # Enabled?
        n132 = event-data() -> ("ModuleID"=w331:i32, "Data"=w330:variant)  [unwired: 1 in]
        n133 = case shown="True" w329 {
          tunnel: [w332 w348] -> w326
          tunnel: w328 -> [w332 w348]
          tunnel: w331 -> [_ w345]
          tunnel: w330 -> [_ w347]
          tunnel: [_ w335] -> w327
          frame False {
          }
          frame True {
            n134 = Variant To Data(type=dbl[] [], Variant=w347) -> (data=w344:dbl[], error out=w340:errorcluster)  [unwired: 1 in]
            n135 = for {
              tunnel: w348 -> [w353] mode=indexing
              tunnel: w345 -> [w351]
              tunnel: [w349] -> w334
              i -> [w349]
              stop <- w350 stop-if-true
              # "Find Bus Index"
              n136 = property class="Bus.lvclass"(reference=w353) -> ("Accessors:EventModuleID"=w352:i32)  [unwired: 1 in, 2 out]
              n137 = Equal?(x=w352, y=w351) -> (x = y?=w350:bool)
            }
            n138 = call <userlib>:"AddError.vi"("Severity"="Critical" ("String"), "Priority"=u8 1, "error in (no error)"=w340) -> ("ErrorArray"=w336:errorcluster[], "error out"=w339:errorcluster)  [unwired: 7 in]
            n139 = call <vilib>:"Clear Errors.vi"("error in (no error)"=w339) -> ()  [unwired: 5 in, 2 out]
            n140 = Bundle(w334, w344) -> (w343:cluster{i32, dbl[]})  [unwired: 1 in]
            n141 = To Variant(anything=w343) -> (Variant=w342:variant)
            n142 = call "Enqueue.vi"("QueName"="BaseVisQue", "Error"=w336, "Data"=w342, "Message"="EvtTimeArray") -> ("Error"=w335:errorcluster[])  [unwired: 7 in]
          }
        }
      }
      event User Event {
        w357 = TRUE  # Enabled?
        n143 = event-data() -> ("ModuleID"=w359:i32, "Data"=w358:variant)  [unwired: 1 in]
        n144 = case shown="True" w357 {
          tunnel: [w360 w376] -> w354
          tunnel: w356 -> [w360 w376]
          tunnel: w359 -> [_ w374]
          tunnel: w358 -> [_ w375]
          tunnel: [_ w364] -> w355
          frame False {
          }
          frame True {
            n145 = Variant To Data(type=T17 {"Status"=""} ("clStatUpdate"), Variant=w375) -> (data=w373:T17, error out=w369:errorcluster)  [unwired: 1 in]
            n146 = for {
              tunnel: w376 -> [w381] mode=indexing
              tunnel: w374 -> [w379]
              tunnel: [w377] -> w363
              i -> [w377]
              stop <- w378 stop-if-true
              # "Find Bus Index"
              n147 = property class="Bus.lvclass"(reference=w381) -> ("Accessors:EventModuleID"=w380:i32)  [unwired: 1 in, 2 out]
              n148 = Equal?(x=w380, y=w379) -> (x = y?=w378:bool)
            }
            n149 = call <userlib>:"AddError.vi"("Severity"="Critical" ("String"), "Priority"=u8 1, "error in (no error)"=w369) -> ("ErrorArray"=w365:errorcluster[], "error out"=w368:errorcluster)  [unwired: 7 in]
            n150 = call <vilib>:"Clear Errors.vi"("error in (no error)"=w368) -> ()  [unwired: 5 in, 2 out]
            n151 = Bundle(w363, "clStatUpdate"=w373) -> (w372:cluster{i32, "clStatUpdate":T17})  [unwired: 1 in]
            n152 = To Variant(anything=w372) -> (Variant=w371:variant)
            n153 = call "Enqueue.vi"("QueName"="BaseVisQue", "Error"=w365, "Data"=w371, "Message"="Status") -> ("Error"=w364:errorcluster[])  [unwired: 7 in]
          }
        }
      }
      event User Event {
        w385 = TRUE  # Enabled?
        n154 = event-data() -> ("ModuleID"=w387:i32, "Data"=w386:variant)  [unwired: 1 in]
        n155 = case shown="True" w385 {
          tunnel: [w388 w404] -> w382
          tunnel: w384 -> [w388 w404]
          tunnel: w387 -> [_ w402]
          tunnel: w386 -> [_ w403]
          tunnel: [_ w392] -> w383
          frame False {
          }
          frame True {
            n156 = Variant To Data(type=T17 {"Status"=""} ("clStatUpdate"), Variant=w403) -> (data=w401:T17, error out=w397:errorcluster)  [unwired: 1 in]
            n157 = for {
              tunnel: w404 -> [w409] mode=indexing
              tunnel: w402 -> [w407]
              tunnel: [w405] -> w391
              i -> [w405]
              stop <- w406 stop-if-true
              # "Find Bus Index"
              n158 = property class="Bus.lvclass"(reference=w409) -> ("Accessors:EventModuleID"=w408:i32)  [unwired: 1 in, 2 out]
              n159 = Equal?(x=w408, y=w407) -> (x = y?=w406:bool)
            }
            n160 = call <userlib>:"AddError.vi"("Severity"="Critical" ("String"), "Priority"=u8 1, "error in (no error)"=w397) -> ("ErrorArray"=w393:errorcluster[], "error out"=w396:errorcluster)  [unwired: 7 in]
            n161 = call <vilib>:"Clear Errors.vi"("error in (no error)"=w396) -> ()  [unwired: 5 in, 2 out]
            n162 = Bundle(w391, "clStatUpdate"=w401) -> (w400:cluster{i32, "clStatUpdate":T17})  [unwired: 1 in]
            n163 = To Variant(anything=w400) -> (Variant=w399:variant)
            n164 = call "Enqueue.vi"("QueName"="BaseVisQue", "Error"=w393, "Data"=w399, "Message"="Status") -> ("Error"=w392:errorcluster[])  [unwired: 7 in]
          }
        }
      }
      event User Event {
        w413 = TRUE  # Enabled?
        n165 = event-data() -> ("ModuleID"=w415:i32, "Data"=w414:variant)  [unwired: 1 in]
        n166 = case shown="True" w413 {
          tunnel: [w416 w432] -> w410
          tunnel: w412 -> [w416 w432]
          tunnel: w415 -> [_ w430]
          tunnel: w414 -> [_ w431]
          tunnel: [_ w420] -> w411
          frame False {
          }
          frame True {
            n167 = Variant To Data(type=T17 {"Status"=""} ("clStatUpdate"), Variant=w431) -> (data=w429:T17, error out=w425:errorcluster)  [unwired: 1 in]
            n168 = for {
              tunnel: w432 -> [w437] mode=indexing
              tunnel: w430 -> [w435]
              tunnel: [w433] -> w419
              i -> [w433]
              stop <- w434 stop-if-true
              # "Find Bus Index"
              n169 = property class="Bus.lvclass"(reference=w437) -> ("Accessors:EventModuleID"=w436:i32)  [unwired: 1 in, 2 out]
              n170 = Equal?(x=w436, y=w435) -> (x = y?=w434:bool)
            }
            n171 = call <userlib>:"AddError.vi"("Severity"="Critical" ("String"), "Priority"=u8 1, "error in (no error)"=w425) -> ("ErrorArray"=w421:errorcluster[], "error out"=w424:errorcluster)  [unwired: 7 in]
            n172 = call <vilib>:"Clear Errors.vi"("error in (no error)"=w424) -> ()  [unwired: 5 in, 2 out]
            n173 = Bundle(w419, "clStatUpdate"=w429) -> (w428:cluster{i32, "clStatUpdate":T17})  [unwired: 1 in]
            n174 = To Variant(anything=w428) -> (Variant=w427:variant)
            n175 = call "Enqueue.vi"("QueName"="BaseVisQue", "Error"=w421, "Data"=w427, "Message"="Status") -> ("Error"=w420:errorcluster[])  [unwired: 7 in]
          }
        }
      }
      event User Event {
        w441 = TRUE  # Enabled?
        n176 = event-data() -> ("ModuleID"=w443:i32, "Data"=w442:variant)  [unwired: 1 in]
        n177 = case shown="True" w441 {
          tunnel: [w444 w460] -> w438
          tunnel: w440 -> [w444 w460]
          tunnel: w443 -> [_ w458]
          tunnel: w442 -> [_ w459]
          tunnel: [_ w448] -> w439
          frame False {
          }
          frame True {
            n178 = Variant To Data(type=T17 {"Status"=""} ("clStatUpdate"), Variant=w459) -> (data=w457:T17, error out=w453:errorcluster)  [unwired: 1 in]
            n179 = for {
              tunnel: w460 -> [w465] mode=indexing
              tunnel: w458 -> [w463]
              tunnel: [w461] -> w447
              i -> [w461]
              stop <- w462 stop-if-true
              # "Find Bus Index"
              n180 = property class="Bus.lvclass"(reference=w465) -> ("Accessors:EventModuleID"=w464:i32)  [unwired: 1 in, 2 out]
              n181 = Equal?(x=w464, y=w463) -> (x = y?=w462:bool)
            }
            n182 = call <userlib>:"AddError.vi"("Severity"="Critical" ("String"), "Priority"=u8 1, "error in (no error)"=w453) -> ("ErrorArray"=w449:errorcluster[], "error out"=w452:errorcluster)  [unwired: 7 in]
            n183 = call <vilib>:"Clear Errors.vi"("error in (no error)"=w452) -> ()  [unwired: 5 in, 2 out]
            n184 = Bundle(w447, "clStatUpdate"=w457) -> (w456:cluster{i32, "clStatUpdate":T17})  [unwired: 1 in]
            n185 = To Variant(anything=w456) -> (Variant=w455:variant)
            n186 = call "Enqueue.vi"("QueName"="BaseVisQue", "Error"=w449, "Data"=w455, "Message"="Status") -> ("Error"=w448:errorcluster[])  [unwired: 7 in]
          }
        }
      }
      event User Event {
        # "Enabled?"
        n187 = event-data() -> ("ModuleID"=w470:i32, "Data"=w469:variant)  [unwired: 1 in]
        n188 = case shown="True" FALSE {
          tunnel: w471 -> [w472 w474]
          tunnel: w470 -> [_ w483]
          tunnel: w469 -> [_ w481]
          tunnel: [_ w478] -> w468
          tunnel: [w472 w474] -> w466
          frame False {
          }
          frame True {
            # "Find Bus Index"
            n189 = for {
              tunnel: w474 -> [w488] mode=indexing
              tunnel: w483 -> [w486]
              tunnel: [w484] -> w482
              i -> [w484]
              stop <- w485 stop-if-true
              n190 = property class="Bus.lvclass"(reference=w488) -> ("Accessors:EventModuleID"=w487:i32)  [unwired: 1 in, 2 out]
              n191 = Equal?(x=w487, y=w486) -> (x = y?=w485:bool)
            }
            n192 = Variant To Data(type=T3 [] ("clEvtReportArray"), Variant=w481) -> (data=w479:T3)  [unwired: 1 in, 1 out]
            n193 = Bundle By Name(cluster=T16 {"BusIndex"=0, "clImpairReportArray"=[]} ("clEvtReportArray"), "BusIndex"=w482, "clImpairReportArray"=w479) -> (w477:T16)
            n194 = local read "QueName"() -> (w473:string)
            n195 = call "Enqueue.vi"("QueName"=w473, "Data"=w477, "Message"="EventReport") -> ("Error"=w478:errorcluster[])  [unwired: 8 in]
          }
        }
      }
      event User Event {
        # "Enabled?"
        n196 = event-data() -> ("ModuleID"=w493:i32, "Data"=w492:variant)  [unwired: 1 in]
        n197 = case shown="True" FALSE {
          tunnel: w494 -> [w495 w497]
          tunnel: w493 -> [_ w506]
          tunnel: w492 -> [_ w504]
          tunnel: [_ w501] -> w491
          tunnel: [w495 w497] -> w489
          frame False {
          }
          frame True {
            # "Find Bus Index"
            n198 = for {
              tunnel: w497 -> [w511] mode=indexing
              tunnel: w506 -> [w509]
              tunnel: [w507] -> w505
              i -> [w507]
              stop <- w508 stop-if-true
              n199 = property class="Bus.lvclass"(reference=w511) -> ("Accessors:EventModuleID"=w510:i32)  [unwired: 1 in, 2 out]
              n200 = Equal?(x=w510, y=w509) -> (x = y?=w508:bool)
            }
            n201 = Variant To Data(type=T5 [] ("dblEventSignalArray"), Variant=w504) -> (data=w502:T5)  [unwired: 1 in, 1 out]
            n202 = Bundle By Name(cluster=T22 {"BusIndex"=0, "dblEventSignalArray"=[]} ("clEvtReportArray"), "BusIndex"=w505, "dblEventSignalArray"=w502) -> (w500:T22)
            n203 = local read "QueName"() -> (w496:string)
            n204 = call "Enqueue.vi"("QueName"=w496, "Data"=w500, "Message"="EventSignal") -> ("Error"=w501:errorcluster[])  [unwired: 8 in]
          }
        }
      }
      event User Event {
        # "Enabled?"
        n205 = event-data() -> ("ModuleID"=w516:i32, "Data"=w515:variant)  [unwired: 1 in]
        n206 = case shown="True" FALSE {
          tunnel: w517 -> [w518 w520]
          tunnel: w516 -> [_ w529]
          tunnel: w515 -> [_ w527]
          tunnel: [_ w524] -> w514
          tunnel: [w518 w520] -> w512
          frame False {
          }
          frame True {
            # "Find Bus Index"
            n207 = for {
              tunnel: w520 -> [w534] mode=indexing
              tunnel: w529 -> [w532]
              tunnel: [w530] -> w528
              i -> [w530]
              stop <- w531 stop-if-true
              n208 = property class="Bus.lvclass"(reference=w534) -> ("Accessors:EventModuleID"=w533:i32)  [unwired: 1 in, 2 out]
              n209 = Equal?(x=w533, y=w532) -> (x = y?=w531:bool)
            }
            n210 = Variant To Data(type=T3 [] ("clEvtReportArray"), Variant=w527) -> (data=w525:T3)  [unwired: 1 in, 1 out]
            n211 = Bundle By Name(cluster=T18 {"BusIndex"=0, "clImpairReportArray"=[]} ("clEvtReportArray"), "BusIndex"=w528, "clImpairReportArray"=w525) -> (w523:T18)
            n212 = local read "QueName"() -> (w519:string)
            n213 = call "Enqueue.vi"("QueName"=w519, "Data"=w523, "Message"="PmuImpairRpt") -> ("Error"=w524:errorcluster[])  [unwired: 8 in]
          }
        }
      }
      event User Event {
        # "Enabled?"
        n214 = event-data() -> ("ModuleID"=w539:i32, "Data"=w538:variant)  [unwired: 1 in]
        n215 = case shown="True" FALSE {
          tunnel: w540 -> [w541 w543]
          tunnel: w539 -> [_ w552]
          tunnel: w538 -> [_ w550]
          tunnel: [_ w547] -> w537
          tunnel: [w541 w543] -> w535
          frame False {
          }
          frame True {
            # "Find Bus Index"
            n216 = for {
              tunnel: w543 -> [w557] mode=indexing
              tunnel: w552 -> [w555]
              tunnel: [w553] -> w551
              i -> [w553]
              stop <- w554 stop-if-true
              n217 = property class="Bus.lvclass"(reference=w557) -> ("Accessors:EventModuleID"=w556:i32)  [unwired: 1 in, 2 out]
              n218 = Equal?(x=w556, y=w555) -> (x = y?=w554:bool)
            }
            n219 = Variant To Data(type=T6 [] ("dblNetworkTime"), Variant=w550) -> (data=w548:T6)  [unwired: 1 in, 1 out]
            n220 = Bundle By Name(cluster=T19 {"BusIndex"=0, "clNetImpairTimeArray"=[]} ("clEvtReportArray"), "BusIndex"=w551, "clNetImpairTimeArray"=w548) -> (w546:T19)
            n221 = local read "QueName"() -> (w542:string)
            n222 = call "Enqueue.vi"("QueName"=w542, "Data"=w546, "Message"="NetImpairTime") -> ("Error"=w547:errorcluster[])  [unwired: 8 in]
          }
        }
      }
      event User Event {
        # "Enabled?"
        n223 = event-data() -> ("ModuleID"=w562:i32, "Data"=w561:variant)  [unwired: 1 in]
        n224 = case shown="True" FALSE {
          tunnel: w563 -> [w564 w566]
          tunnel: w562 -> [_ w575]
          tunnel: w561 -> [_ w573]
          tunnel: [_ w570] -> w560
          tunnel: [w564 w566] -> w558
          frame False {
          }
          frame True {
            # "Find Bus Index"
            n225 = for {
              tunnel: w566 -> [w580] mode=indexing
              tunnel: w575 -> [w578]
              tunnel: [w576] -> w574
              i -> [w576]
              stop <- w577 stop-if-true
              n226 = property class="Bus.lvclass"(reference=w580) -> ("Accessors:EventModuleID"=w579:i32)  [unwired: 1 in, 2 out]
              n227 = Equal?(x=w579, y=w578) -> (x = y?=w577:bool)
            }
            n228 = Variant To Data(type=T7 [] ("dblPktLoss"), Variant=w573) -> (data=w571:T7)  [unwired: 1 in, 1 out]
            n229 = Bundle By Name(cluster=T20 {"BusIndex"=0, "clNetPktLoss"=[]} ("clEvtReportArray"), "BusIndex"=w574, "clNetPktLoss"=w571) -> (w569:T20)
            n230 = local read "QueName"() -> (w565:string)
            n231 = call "Enqueue.vi"("QueName"=w565, "Data"=w569, "Message"="NetPktLoss") -> ("Error"=w570:errorcluster[])  [unwired: 8 in]
          }
        }
      }
      event User Event {
        # "Enabled?"
        n232 = event-data() -> ("ModuleID"=w585:i32, "Data"=w584:variant)  [unwired: 1 in]
        n233 = case shown="True" FALSE {
          tunnel: w586 -> [w587 w589]
          tunnel: w585 -> [_ w598]
          tunnel: w584 -> [_ w596]
          tunnel: [_ w593] -> w583
          tunnel: [w587 w589] -> w581
          frame False {
          }
          frame True {
            # "Find Bus Index"
            n234 = for {
              tunnel: w589 -> [w603] mode=indexing
              tunnel: w598 -> [w601]
              tunnel: [w599] -> w597
              i -> [w599]
              stop <- w600 stop-if-true
              n235 = property class="Bus.lvclass"(reference=w603) -> ("Accessors:EventModuleID"=w602:i32)  [unwired: 1 in, 2 out]
              n236 = Equal?(x=w602, y=w601) -> (x = y?=w600:bool)
            }
            n237 = Variant To Data(type=T8 [] ("ui32FlagImpairmentArray"), Variant=w596) -> (data=w594:T8)  [unwired: 1 in, 1 out]
            n238 = Bundle By Name(cluster=T21 {"BusIndex"=0, "FlagImpairArray"=[]} ("clEvtReportArray"), "BusIndex"=w597, "FlagImpairArray"=w594) -> (w592:T21)
            n239 = local read "QueName"() -> (w588:string)
            n240 = call "Enqueue.vi"("QueName"=w588, "Data"=w592, "Message"="FlagImpair") -> ("Error"=w593:errorcluster[])  [unwired: 8 in]
          }
        }
      }
      event "btnStop": Value Change {
        n241 = event-data() -> ()  [unwired: 1 in, 1 out]
        n242 = call "ObtainRequestEvents.vi"() -> ("Error"=w614:errorcluster[], "clRequestEvents"=w611:T9)  [unwired: 10 in]
        n243 = Unbundle By Name(w611) -> ("StopRequest"=w612:refnum<user-event>)
        n244 = Generate User Event(priority (normal)=usereventprio."high priority", user event=w612, event data cluster=T23 {"BusIndex"=0, "Data"=variant} ("event data")) -> (error out=w613:errorcluster)  [unwired: 1 in, 1 out]
        n245 = call <userlib>:"AddError.vi"("Severity"="Fatal" ("String"), "Priority"=u8 0, "ErrorArray"=w614, "error in (no error)"=w613) -> ("ErrorArray"=w610:errorcluster[], "error out"=w607:errorcluster)  [unwired: 6 in]
        n246 = call <vilib>:"Clear Errors.vi"("error in (no error)"=w607) -> ()  [unwired: 5 in, 2 out]
      }
    }
    n247 = local read "QueName"() -> (w269:string)
    n248 = call "EnqueError.vi"("QueName"=w269, "Error"=w274) -> ("Error"=w273:errorcluster[])  [unwired: 9 in]
  }
  n249 = Build Array (concatenate)(w27, w28) -> (w2:errorcluster[])
  "ErrorArray" <- w2
  n250 = Index Array(array=w2) -> (element=w1:errorcluster)  [unwired: 1 in]
  n251 = invoke class="VI" method="FP.Close"(error in=w1) -> ()  [unwired: 2 in, 3 out]
